vi "ConfigInstr.vi"(6 "InstrumentName":string, 7 "VisaRessIn":refnum<visa-resource-name>, 8 "error in (no error)":errorcluster caption="entrée d'erreur (pas d'erreur)", 9 "FirstClassInst":bool, 10 "Function":string, 11 "GenData In":refnum<class "DAQ6363.lvclass"> caption="DNL_LabVIEW Object in") -> (0 "error out":errorcluster caption="sortie d'erreur", 3 "GenData Out":refnum<class "DAQ6363.lvclass"> caption="DNL_LabVIEW Object out")   [LabVIEW 2019, in "DAQ6363.lvclass"]
uses:
  DAQ6363.lvclass
  C:/Programmes Labview/LabScanV1A/DevicesClass/BaseDevice/BaseDevice.lvclass
  DAQ6363_Func.ctl
  DAQ6363.lvclass/DAQ6363.ctl
  BaseDevice/BaseDevice.lvclass/BaseDevice.ctl
  BaseDevice/Accessor/SetShowInstrNm.vi
  BaseDevice/Accessor/SetInstrParam.vi
panel:
  in  "Class_Func":T1
  out "VisaRessOut":refnum<visa-resource-name>
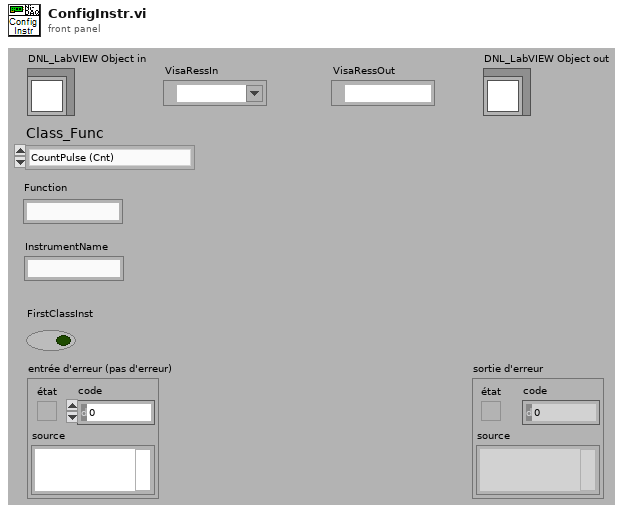
[diagram p1: front panel]
types:
  T1 = typedef "DAQ6363.lvclass/DAQ6363_Func.ctl" = enum16{"CountPulse (Cnt)", "Rabi (Tau)", "MWtoLaserDelay (us)", "APDGate (us)", "PulsedODMR (Pulses)", "PulsedODMR_AWG (Pulses)", "DiffODMRSglPulseAWG (Pulses)", "DiffPulsedODMR_AWG (Pulses)", "GatedPulseCount (Pulses)", "DiffPulsedODMR (Pulses)"}
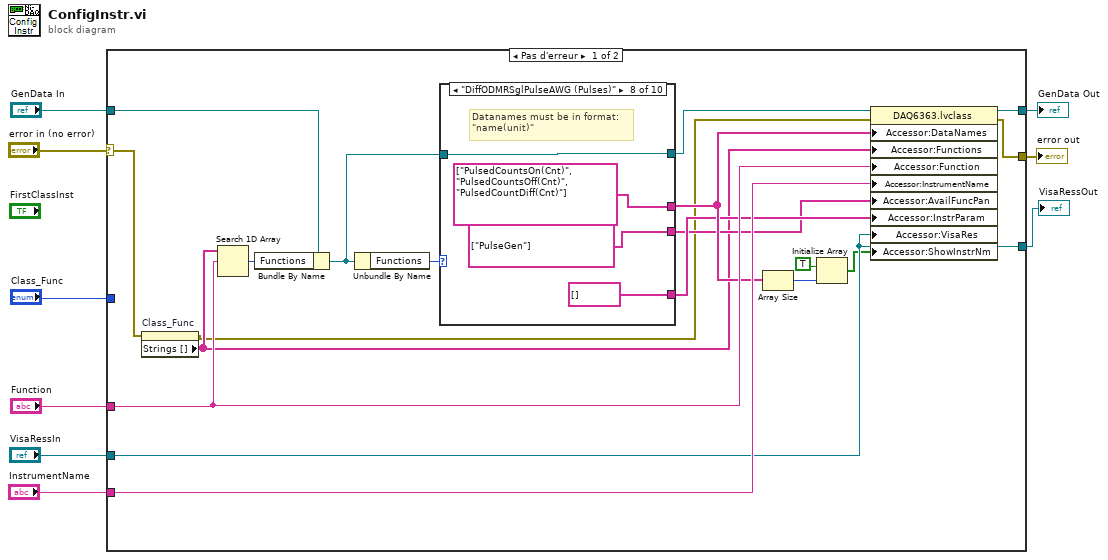
[diagram p0: block diagram]
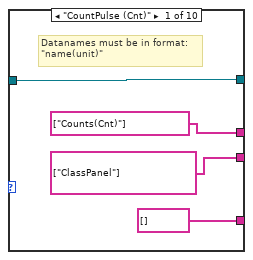
[diagram p2: hidden frame]
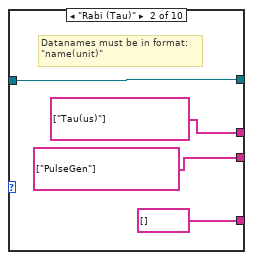
[diagram p3: hidden frame]
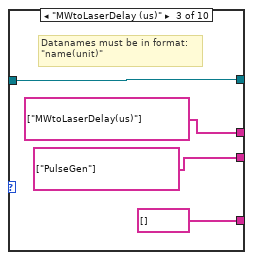
[diagram p4: hidden frame]
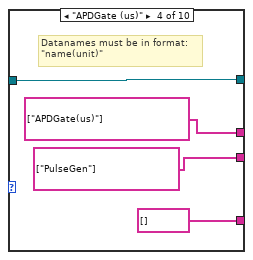
[diagram p5: hidden frame]
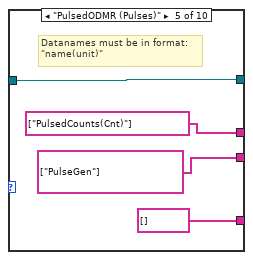
[diagram p6: hidden frame]
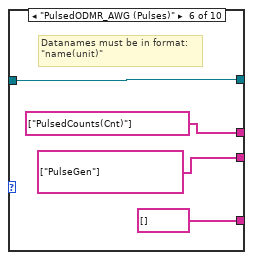
[diagram p7: hidden frame]
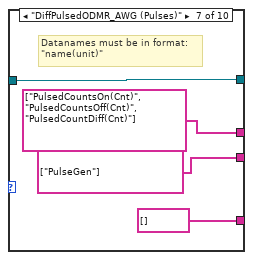
[diagram p8: hidden frame]
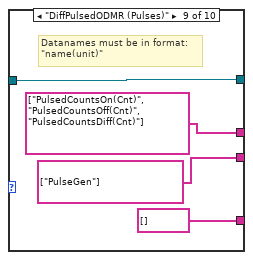
[diagram p9: hidden frame]
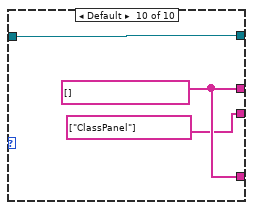
[diagram p10: hidden frame]
diagram:
  n1 = case shown="Pas d'erreur" "error in (no error)" {
    selector: "error in (no error)" -> [w11 w69]
    tunnel: [w28 w69] -> w8
    tunnel: "GenData In" -> [w24 w68]
    tunnel: [w27 w68] -> w6
    tunnel: "Class_Func" -> [_ _]
    tunnel: "Function" -> [w21 _]
    tunnel: "InstrumentName" -> [w20 _]
    tunnel: "VisaRessIn" -> [w19 _]
    tunnel: [w19 _] -> w1
    frame No Error {
      n2 = property on="Class_Func" class="Énum (strict)"(error in=w11) -> (error out=w10:errorcluster, "Strings []"=w12:string[])  [unwired: 1 in, 1 out]
      n3 = Search 1D Array(1D array=w12, element=w21) -> (index of element=w25:i32)  [unwired: 1 in]
      n4 = Bundle By Name(cluster=w24, "Functions"=w25) -> (w23:refnum<class "DAQ6363.lvclass">)
      n5 = Unbundle By Name(w23) -> ("Functions"=w26:T1)
      n6 = case shown="\"DiffODMRSglPulseAWG (Pulses)\"" w26 {
        tunnel: [string[] ["Counts(Cnt)"] string[] ["Tau(us)"] string[] ["MWtoLaserDelay(us)"] string[] ["APDGate(us)"] string[] ["PulsedCounts(Cnt)"] string[] ["PulsedCounts(Cnt)"] string[] ["PulsedCountsOn(Cnt)", "PulsedCountsOff(Cnt)", "PulsedCountDiff(Cnt)"] string[] ["PulsedCountsOn(Cnt)", "PulsedCountsOff(Cnt)", "PulsedCountDiff(Cnt)"] string[] ["PulsedCountsOn(Cnt)", "PulsedCountsOff(Cnt)", "PulsedCountsDiff(Cnt)"] w66] -> w16
        tunnel: w23 -> [w32 w36 w40 w44 w48 w52 w56 w60 w64 w67]
        tunnel: [w32 w36 w40 w44 w48 w52 w56 w60 w64 w67] -> w22
        tunnel: [string[] [] string[] [] string[] [] string[] [] string[] [] string[] [] string[] [] string[] [] string[] [] w66] -> w14
        tunnel: [string[] ["ClassPanel"] string[] ["PulseGen"] string[] ["PulseGen"] string[] ["PulseGen"] string[] ["PulseGen"] string[] ["PulseGen"] string[] ["PulseGen"] string[] ["PulseGen"] string[] ["PulseGen"] string[] ["ClassPanel"]] -> w13
        frame "CountPulse (Cnt)" {
          # "Datanames must be in format:\n\"name(unit)\""
        }
        frame "Rabi (Tau)" {
          # "Datanames must be in format:\n\"name(unit)\""
        }
        frame "MWtoLaserDelay (us)" {
          # "Datanames must be in format:\n\"name(unit)\""
        }
        frame "APDGate (us)" {
          # "Datanames must be in format:\n\"name(unit)\""
        }
        frame "PulsedODMR (Pulses)" {
          # "Datanames must be in format:\n\"name(unit)\""
        }
        frame "PulsedODMR_AWG (Pulses)" {
          # "Datanames must be in format:\n\"name(unit)\""
        }
        frame "DiffPulsedODMR_AWG (Pulses)" {
          # "Datanames must be in format:\n\"name(unit)\""
        }
        frame "DiffODMRSglPulseAWG (Pulses)" {
          # "Datanames must be in format:\n\"name(unit)\""
        }
        frame "DiffPulsedODMR (Pulses)" {
          # "Datanames must be in format:\n\"name(unit)\""
        }
        frame Default {
          w66 = string[] []
        }
      }
      n7 = Array Size(array=w16) -> (size(s)=w18:i32)
      n8 = Initialize Array(TRUE, w18) -> (w15:bool[])
      n9 = property class="DAQ6363.lvclass"(reference=w22, error in=w10, "Accessor:DataNames"=w16, "Accessor:Functions"=w12, "Accessor:Function"=w21, "Accessor:InstrumentName"=w20, "Accessor:AvailFuncPan"=w13, "Accessor:InstrParam"=w14, "Accessor:VisaRes"=w19, "Accessor:ShowInstrNm"=w15) -> (reference out=w27:refnum<class "DAQ6363.lvclass">, error out=w28:errorcluster)
    }
    frame Error {
    }
  }
  "error out" <- w8
  "GenData Out" <- w6
  "VisaRessOut" <- w1
